vi "Configure LEDs.vi"(0 "niUsrpRio Session":T2={"FPGA Interface"=refnum, "RIO Interface Number"=0, "Data Clock Rate"=0, "FPGA Data Clock Rate"=0, "Global Settings Register Bus"=refnum, "Radio 0 Settings Register Bus"=refnum, "Radio 1 Settings Register Bus"=refnum, "Radio Settings Bus Semaphore"=refnum, "DB Queues"=[], "Characterization Data Valid?"=FALSE, "EEPROM Header"={"Checksum"=0, "Product Code"=0, "Hardware Current Version"=0, "Hardware Oldest Compatible Version"=0, "EEPROM Map Current Version"=0, "EEPROM Map Oldest Compatible Version"=0, "User Password"="", "Pointer to Factory Header"=0, "Pointer to User Header"=0, "Recommended Interval"=0, "Number of Reserved Bytes"=9, "Number of Daughterboards"=0, "Daughterboard IDs"=[], "Daughterboard Serial Numbers"=[]}, "Device Data Header"={"Checksum"=0, "Number of Channels"=0, "Number of Gain Settings"=[], "Pointer to Characterization Data"=[], "Number of Reserved Bytes"=27, "Number of Frequencies"=[]}, "EEPROM Characterization Header"={"Checksum"=0, "Date"=timestamp(0 s since 1904-01-01), "Temperature"=0.0, "Misc. Info"="", "Pointer to Device Data Header"=0, "Number of Reserved Bytes"=28}, "Characterization Data"=[], "FPGA Current Version"=0, "FPGA Oldest Compatible Version"=0, "Fixed Logic Current Version"=0, "Fixed Logic Oldest Compatible Version"=0, "FPGA Radio Settings Bus Current Version"=0, "FPGA Radio Settings Bus Oldest Compatible Version"=0, "FPGA Board Config Current Version"=0, "FPGA Board Config Oldest Compatible Version"=0, "Daughterboard Clock Rate"=0, "daughterboard configuration session handles"=[]} {"Daughterboard Clock Rate" format="%#.3pHz"; "FPGA Data Clock Rate" format="%#.3pHz"; "Data Clock Rate" format="%#.3pHz"; "Characterization Data"."Frequencies [Hz]" format="%#_6p"; "EEPROM Characterization Header"."Pointer to Device Data Header" format="%x"; "EEPROM Characterization Header"."Checksum" format="%x"; "Device Data Header"."Pointer to Characterization Data" format="%x"; "Device Data Header"."Checksum" format="%x"; "EEPROM Header"."Pointer to User Header" format="%x"; "EEPROM Header"."Pointer to Factory Header" format="%x"; "EEPROM Header"."Product Code" format="%x"; "EEPROM Header"."Checksum" format="%x"}, 1 "scope":string(combo), 5 "channel configurations":T1(array[cluster]) {"channel configuration"."frequency" format="%#.3pHz"; "channel configuration"."lo frequency" format="%#.3pHz"; "channel configuration"."level" format="%#_gdBm"}, 11 "error in":errorcluster) -> (4 "niUsrpRio Session (out)":T2={"FPGA Interface"=refnum, "RIO Interface Number"=0, "Data Clock Rate"=0, "FPGA Data Clock Rate"=0, "Global Settings Register Bus"=refnum, "Radio 0 Settings Register Bus"=refnum, "Radio 1 Settings Register Bus"=refnum, "Radio Settings Bus Semaphore"=refnum, "DB Queues"=[], "Characterization Data Valid?"=FALSE, "EEPROM Header"={"Checksum"=0, "Product Code"=0, "Hardware Current Version"=0, "Hardware Oldest Compatible Version"=0, "EEPROM Map Current Version"=0, "EEPROM Map Oldest Compatible Version"=0, "User Password"="", "Pointer to Factory Header"=0, "Pointer to User Header"=0, "Recommended Interval"=0, "Number of Reserved Bytes"=9, "Number of Daughterboards"=0, "Daughterboard IDs"=[], "Daughterboard Serial Numbers"=[]}, "Device Data Header"={"Checksum"=0, "Number of Channels"=0, "Number of Gain Settings"=[], "Pointer to Characterization Data"=[], "Number of Reserved Bytes"=27, "Number of Frequencies"=[]}, "EEPROM Characterization Header"={"Checksum"=0, "Date"=timestamp(0 s since 1904-01-01), "Temperature"=0.0, "Misc. Info"="", "Pointer to Device Data Header"=0, "Number of Reserved Bytes"=28}, "Characterization Data"=[], "FPGA Current Version"=0, "FPGA Oldest Compatible Version"=0, "Fixed Logic Current Version"=0, "Fixed Logic Oldest Compatible Version"=0, "FPGA Radio Settings Bus Current Version"=0, "FPGA Radio Settings Bus Oldest Compatible Version"=0, "FPGA Board Config Current Version"=0, "FPGA Board Config Oldest Compatible Version"=0, "Daughterboard Clock Rate"=0, "daughterboard configuration session handles"=[]} {"Daughterboard Clock Rate" format="%#.3pHz"; "FPGA Data Clock Rate" format="%#.3pHz"; "Data Clock Rate" format="%#.3pHz"; "Characterization Data"."Frequencies [Hz]" format="%#_6p"; "EEPROM Characterization Header"."Pointer to Device Data Header" format="%x"; "EEPROM Characterization Header"."Checksum" format="%x"; "Device Data Header"."Pointer to Characterization Data" format="%x"; "Device Data Header"."Checksum" format="%x"; "EEPROM Header"."Pointer to User Header" format="%x"; "EEPROM Header"."Pointer to Factory Header" format="%x"; "EEPROM Header"."Product Code" format="%x"; "EEPROM Header"."Checksum" format="%x"}, 15 "error out":errorcluster)   [LabVIEW 2020]
uses:
  <instrlib>/niUsrpRio/Config/v1/Host/Public/niUsrpRio Session.ctl
  <instrlib>/_niInstr/Register Bus/v0/Host/Public/Register Bus Session.ctl
  <instrlib>/_niInstr/Register Bus/v0/Host/Private/Session Data.ctl
  <instrlib>/niUsrpRio/Config/v1/Host/Private/DB Queue Reference.ctl
  <instrlib>/niUsrpRio/Config/v1/Host/Private/Daughterboard Data.ctl
  <instrlib>/niUsrpRio/Config/v1/Host/Private/ATR state data.ctl
  <instrlib>/niUsrpRio/Config/v1/Host/Private/Antenna Configuration.ctl
  <instrlib>/niUsrpRio/Config/v1/Host/Private/CPLD Power Mode.ctl
  <instrlib>/niUsrpRio/Config/v1/Host/Public/EEPROM Header.ctl
  <instrlib>/niUsrpRio/Config/v1/Host/Public/EEPROM Device Data Header.ctl
  <instrlib>/niUsrpRio/Config/v1/Host/Public/EEPROM Characterization Header.ctl
  <instrlib>/niUsrpRio/Config/v1/Host/Public/Characterization Data.ctl
  <instrlib>/niUsrpRio/Config/v1/Host/Public/IQ Imbalance.ctl
  Streaming Xvcr FPGA Ref.ctl
  <vilib>/Utility/error.llb/Error Cluster From Error Code.vi
  <vilib>/rvi/errors/niLvFpgaAdjustHostInterfaceError.vi
  <vilib>/rvi/interface/nirviReadWriteControl/nirviReadWriteControl.xnode
  <vilib>/rvi/interface/Simulation/niFpgaSimulationCallBeginRW.vi
  NiFpgaLv.dll
  <instrlib>/niUsrpRio/Config/v1/Host/niUsrpRio Config v1 Host.lvlib
  <instrlib>/_niInstr/Register Bus/v0/Host/niInstr Register Bus v0 Host.lvlib
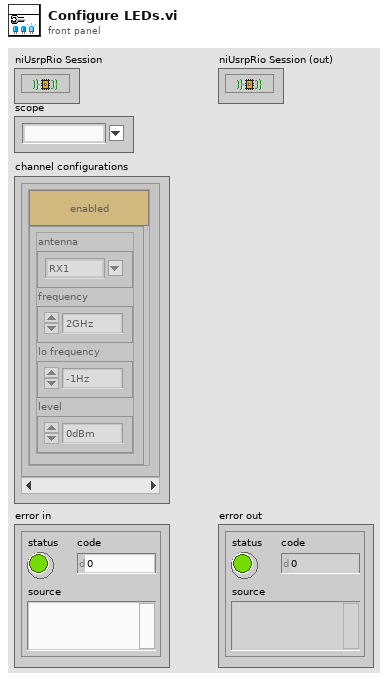
[diagram p1: front panel]
types:
  T1 = cluster{"channel enable":bool, "channel configuration":cluster{"antenna":string, "frequency":dbl, "lo frequency":dbl, "level":dbl}}[]
  T2 = typedef "niUsrpRio Config v1 Host.lvlib/niUsrpRio Session.ctl" = cluster{"FPGA Interface":refnum<k20>, "RIO Interface Number":u32, "Data Clock Rate":u32, "FPGA Data Clock Rate":u32, "Global Settings Register Bus":T3, "Radio 0 Settings Register Bus":T3, "Radio 1 Settings Register Bus":T3, "Radio Settings Bus Semaphore":T4, "DB Queues":T5[], "Characterization Data Valid?":bool, "EEPROM Header":T6, "Device Data Header":T7, "EEPROM Characterization Header":T8, "Characterization Data":T9[], "FPGA Current Version":u32, "FPGA Oldest Compatible Version":u32, "Fixed Logic Current Version":u32, "Fixed Logic Oldest Compatible Version":u32, "FPGA Radio Settings Bus Current Version":u32, "FPGA Radio Settings Bus Oldest Compatible Version":u32, "FPGA Board Config Current Version":u32, "FPGA Board Config Oldest Compatible Version":u32, "Daughterboard Clock Rate":u32, "daughterboard configuration session handles":u64[]}
  T3 = typedef "niInstr Register Bus v0 Host.lvlib/Register Bus Session.ctl" = refnum<queue>
  T4 = typedef "Semaphore RefNum" = refnum<k1>
  T5 = typedef "niUsrpRio Config v1 Host.lvlib/DB Queue Reference.ctl" = refnum<queue>
  T6 = typedef "niUsrpRio Config v1 Host.lvlib/EEPROM Header.ctl" = cluster{"Checksum":u32, "Product Code":u16, "Hardware Current Version":u16, "Hardware Oldest Compatible Version":u16, "EEPROM Map Current Version":u16, "EEPROM Map Oldest Compatible Version":u16, "User Password":string, "Pointer to Factory Header":u32, "Pointer to User Header":u32, "Recommended Interval":u16, "Number of Reserved Bytes":i32, "Number of Daughterboards":u8, "Daughterboard IDs":u16[], "Daughterboard Serial Numbers":string[]}
  T7 = typedef "niUsrpRio Config v1 Host.lvlib/EEPROM Device Data Header.ctl" = cluster{"Checksum":u32, "Number of Channels":u8, "Number of Gain Settings":u16[], "Pointer to Characterization Data":u32[], "Number of Reserved Bytes":i32, "Number of Frequencies":u16[]}
  T8 = typedef "niUsrpRio Config v1 Host.lvlib/EEPROM Characterization Header.ctl" = cluster{"Checksum":u32, "Date":timestamp, "Temperature":sgl, "Misc. Info":string, "Pointer to Device Data Header":u32, "Number of Reserved Bytes":i32}
  T9 = typedef "niUsrpRio Config v1 Host.lvlib/Characterization Data.ctl" = cluster{"Gains[dB]":dbl[], "Frequencies [Hz]":dbl[], "IQ Imbalance Table":T10[], "Measured Gains[dB]":dbl[][]}
  T10 = typedef "niUsrpRio Config v1 Host.lvlib/IQ Imbalance.ctl" = cluster{"Gain Imbalance [linear]":dbl, "Phase Imbalance [radians]":dbl, "Offset":cdb}
  T11 = typedef "Streaming Xvcr FPGA Ref.ctl" = refnum<k20>
  T12 = enum16{"None", "RF 0/RX 1", "RF 0/RX 2", "RF 1/RX 1", "RF 1/RX 2"}
  T13 = cluster{"antenna":string, "frequency":dbl, "lo frequency":dbl, "level":dbl}
  T14 = typedef "niUsrpRio Config v1 Host.lvlib/Device Subfunction.ctl" = enum16{"rx", "tx", "all"}
  T15 = typedef "niUsrpRio Config v1 Host.lvlib/RF Channel 2.ctl" = enum16{"0", "1", "2", "3", "All"}
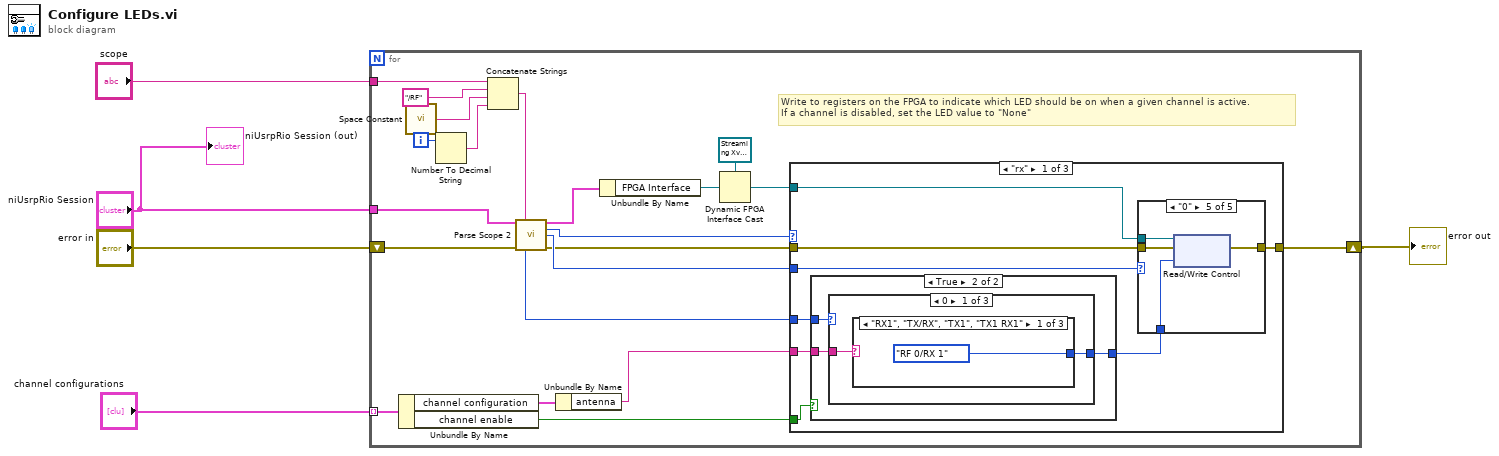
[diagram p0: block diagram]
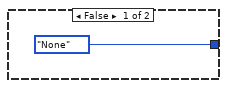
[diagram p2: hidden frame]
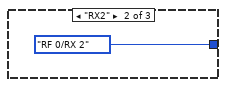
[diagram p3: hidden frame]
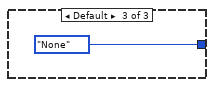
[diagram p4: hidden frame]
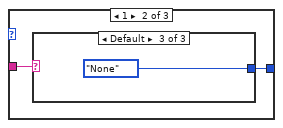
[diagram p5: hidden frame]
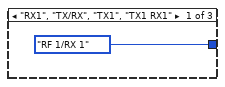
[diagram p6: hidden frame]
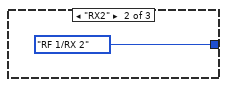
[diagram p7: hidden frame]
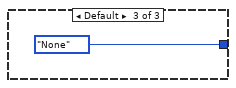
[diagram p8: hidden frame]
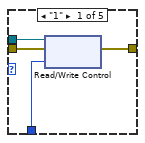
[diagram p9: hidden frame]
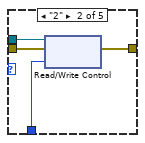
[diagram p10: hidden frame]
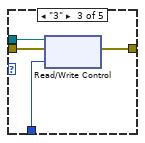
[diagram p11: hidden frame]
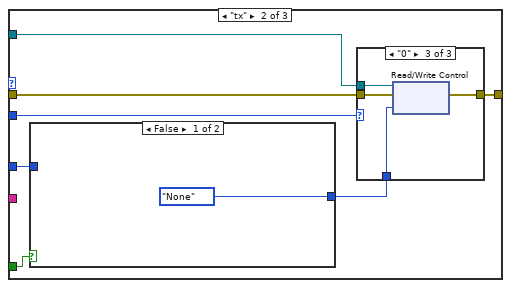
[diagram p13: hidden frame]
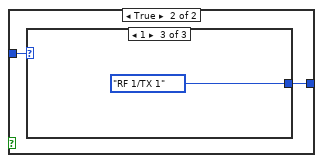
[diagram p14: hidden frame]
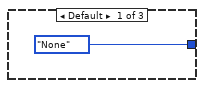
[diagram p15: hidden frame]
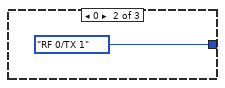
[diagram p16: hidden frame]
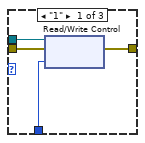
[diagram p17: hidden frame]
diagram:
  n1 = for {
    tunnel: "scope" -> [w26]
    tunnel: "channel configurations" -> [w21] mode=indexing
    tunnel: "niUsrpRio Session" -> [w11]
    shift-right: [w9] -> w1
    shift-left: "error in" -> [w10]
    i -> [w24]
    # "Write to registers on the FPGA to indicate which LED should be on when a given channel is active.\nIf a channel is disabled, set the LED value to \"None\""
    n2 = Unbundle By Name(w21) -> ("channel configuration"=w20:T13, "channel enable"=w7:bool)
    n3 = call <vilib>:"Space Constant.vi"() -> ("String"=w22:string)
    n4 = Number To Decimal String(number=w24) -> (decimal integer string=w25:string)  [unwired: 1 in]
    n5 = Concatenate Strings(w26, "/RF" ("string"), w22, w25) -> (w6:string)
    n6 = call <instrlib>:"Parse Scope 2.vi"("niUsrpRio Session"=w11, "scope"=w6, "error in"=w10) -> ("niUsrpRio Session (out)"=w13:T2, "Device Subfunction"=w12:T14, "Device Subfunction Channel"=w18:T15, "daughterboard index"=w19:u32, "error out"=w14:errorcluster)  [unwired: 4 in, 4 out]
    n7 = Unbundle By Name(w20) -> ("antenna"=w8:string)
    n8 = Unbundle By Name(w13) -> ("FPGA Interface"=w15:refnum<k20>)
    n9 = Dynamic FPGA Interface Cast(Session In=T11 refnum ("FPGA VI Reference Out"), Type=w15) -> (Session Out=w17:T11)
    n10 = case shown="\"rx\"" w12 {
      tunnel: w17 -> [w32 w71 _]
      tunnel: [w34 w73 w89] -> w9
      tunnel: w14 -> [w33 w72 w89]
      tunnel: w18 -> [w29 w69 _]
      tunnel: w19 -> [w31 w70 _]
      tunnel: w8 -> [w28 _ _]
      tunnel: w7 -> [w27 w67 _]
      frame "rx" {
        n11 = case shown="True" w27 {
          tunnel: w31 -> [_ w38]
          tunnel: [T12."None" ("rx 0.led") w37] -> w30
          tunnel: w28 -> [_ w36]
          frame False {
          }
          frame True {
            n12 = case shown="0" w38 {
              tunnel: [w40 w45 T12."None" ("rx 0.led")] -> w37
              tunnel: w36 -> [w39 w44 _]
              frame 0 {
                n13 = case shown="\"RX1\", \"TX/RX\", \"TX1\", \"TX1 RX1\"" w39 {
                  tunnel: [T12."RF 0/RX 1" ("rx 0.led") T12."RF 0/RX 2" ("rx 0.led") T12."None" ("rx 0.led")] -> w40
                  frame "RX1", "TX/RX", "TX1", "TX1 RX1" {
                  }
                  frame "RX2" {
                  }
                  frame Default {
                  }
                }
              }
              frame 1 {
                n14 = case shown="Default" w44 {
                  tunnel: [T12."RF 1/RX 1" ("rx 0.led") T12."RF 1/RX 2" ("rx 0.led") T12."None" ("rx 0.led")] -> w45
                  frame "RX1", "TX/RX", "TX1", "TX1 RX1" {
                  }
                  frame "RX2" {
                  }
                  frame Default {
                  }
                }
              }
              frame Default {
              }
            }
          }
        }
        n15 = case shown="\"0\"" w29 {
          tunnel: [w53 w57 w61 w62 w66] -> w34
          tunnel: w33 -> [w52 w56 w60 w62 w65]
          tunnel: w32 -> [w51 w55 w59 _ w64]
          tunnel: w30 -> [w50 w54 w58 _ w63]
          frame "1" {
            n16 = xnode "Read/Write Control"("FPGA VI Reference In"=w51, "error in"=w52, "rx 1.led"=w50) -> ("error out"=w53:errorcluster)  [unwired: 1 out]
          }
          frame "2" {
            n17 = xnode "Read/Write Control"("FPGA VI Reference In"=w55, "error in"=w56, "rx 2.led"=w54) -> ("error out"=w57:errorcluster)  [unwired: 1 out]
          }
          frame "3" {
            n18 = xnode "Read/Write Control"("FPGA VI Reference In"=w59, "error in"=w60, "rx 3.led"=w58) -> ("error out"=w61:errorcluster)  [unwired: 1 out]
          }
          frame Default {
          }
          frame "0" {
            n19 = xnode "Read/Write Control"("FPGA VI Reference In"=w64, "error in"=w65, "rx 0.led"=w63) -> ("error out"=w66:errorcluster)  [unwired: 1 out]
          }
        }
      }
      frame "tx" {
        n20 = case shown="False" w67 {
          tunnel: w70 -> [_ w76]
          tunnel: [enum16{"None", "RF 0/TX 1", "RF 1/TX 1"}."None" ("tx 0.led") w75] -> w68
          frame False {
          }
          frame True {
            n21 = case shown="1" w76 {
              tunnel: [enum16{"None", "RF 0/TX 1", "RF 1/TX 1"}."None" ("tx 0.led") enum16{"None", "RF 0/TX 1", "RF 1/TX 1"}."RF 0/TX 1" ("tx 0.led") enum16{"None", "RF 0/TX 1", "RF 1/TX 1"}."RF 1/TX 1" ("tx 0.led")] -> w75
              frame Default {
              }
              frame 0 {
              }
              frame 1 {
              }
            }
          }
        }
        n22 = case shown="\"0\"" w69 {
          tunnel: [w83 w84 w88] -> w73
          tunnel: w72 -> [w82 w84 w87]
          tunnel: w71 -> [w81 _ w86]
          tunnel: w68 -> [w80 _ w85]
          frame "1" {
            n23 = xnode "Read/Write Control"("FPGA VI Reference In"=w81, "error in"=w82, "tx 1.led"=w80) -> ("error out"=w83:errorcluster)  [unwired: 1 out]
          }
          frame Default {
          }
          frame "0" {
            n24 = xnode "Read/Write Control"("FPGA VI Reference In"=w86, "error in"=w87, "tx 0.led"=w85) -> ("error out"=w88:errorcluster)  [unwired: 1 out]
          }
        }
      }
      frame Default {
      }
    }
  }
  "error out" <- w1
  "niUsrpRio Session (out)" <- "niUsrpRio Session"
